vi "首行行号.vi"(10 "原始行":dbl, 11 "保留行数":dbl) -> (3 "新行":dbl)   [LabVIEW 2019]
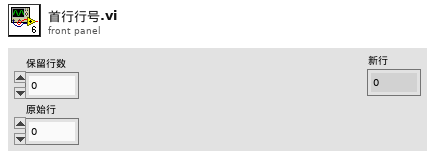
[diagram p1: front panel]
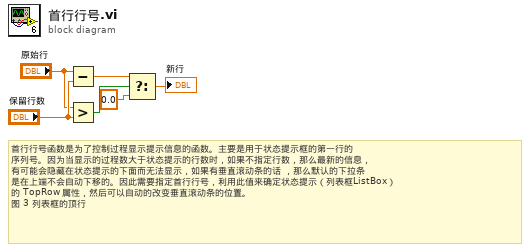
[diagram p0: block diagram]
diagram:
  # "首行行号函数是为了控制过程显示提示信息的函数。主要是用于状态提示框的第一行的\n序列号。因为当显示的过程数大于状态提示的行数时，如果不指定行数，那么最新的信息，\n有可能会隐藏在状态提示的下面而无法显示，如果有垂直滚动条的话 ，那么默认的下拉条\n是在上端不会自动下移的。因此需要指定首行行号，利用此值来确定状态提示（列表框ListBox）\n的 TopRow 属性，然后可以自动的改变垂直滚动条的位置。\n图 3 列表框的顶行"
  n1 = Subtract(x="原始行", y="保留行数") -> (x-y=w5:dbl)
  n2 = Greater?(x="原始行", y="保留行数") -> (0:w6:bool)
  n3 = Select(t=w5, s=w6, f=0.0) -> (s? t:f=→"新行":dbl)
